vi "globe.vi"() -> ()   [LabVIEW 2020]
panel:
  out "总线利用率视图已打开":bool
  in  "通道波特率":u32
  in  "总线比特数":u64
  out "总线错误帧数":u32
  out "接收帧数":u32
  out "发送帧数":u32
  out "ret_ok":bool
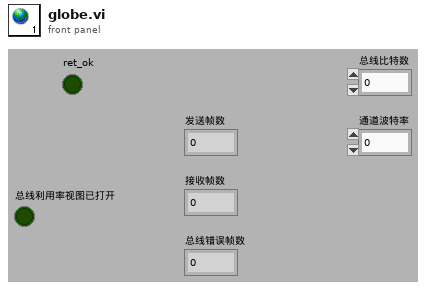
[diagram p1: front panel]
diagram:
